vi "read_pbot_temperature.vi"(11 "Equip_Data":T1 {"h5File_refOut" format="%.0x"; "h5File_dsetOut" format="%.0x"}) -> (0 "error out":errorcluster, 3 "Temperature":dbl)   [LabVIEW 2015]
uses:
  controls/Equip_Data.ctl
  <vilib>/Utility/miscctls.llb/LV3DPointTypeDef.ctl
  controls/startScanData.ctl
  controls/scanInstrumentInfo.ctl
  <vilib>/addons/h5labview2/base/hid_t.ctl
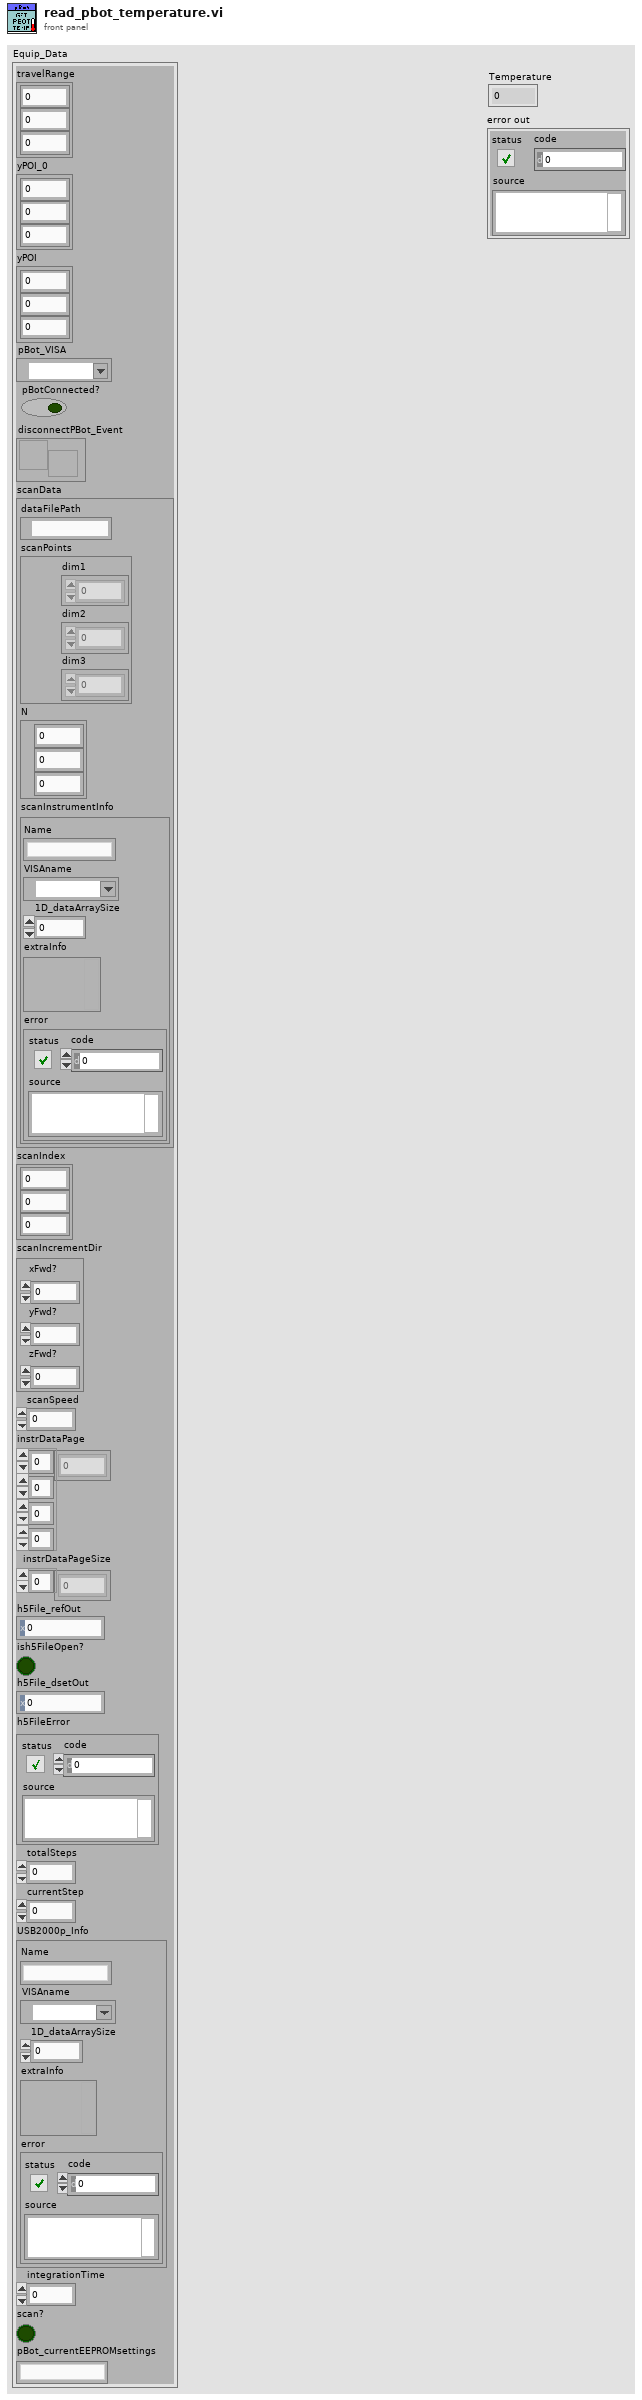
[diagram p1: front panel]
types:
  T1 = typedef "Equip_Data.ctl" = cluster{"travelRange":T2, "yPOI_0":T2, "yPOI":T2, "pBot_VISA":refnum<visa-resource-name>, "pBotConnected?":bool, "disconnectPBot_Event":refnum<user-event>, "scanData":T3, "scanIndex":cluster{"X":u16, "Y":u16, "Z":u16}, "scanIncrementDir":cluster{"xFwd?":i16, "yFwd?":i16, "zFwd?":i16}, "scanSpeed":u16, "instrDataPage":dbl[][][][], "instrDataPageSize":i32[], "h5File_refOut":T5, "ish5FileOpen?":bool, "h5File_dsetOut":T5, "h5FileError":errorcluster, "totalSteps":u32, "currentStep":u32, "USB2000p_Info":T4, "integrationTime":u32, "scan?":bool, "pBot_currentEEPROMsettings":string}
  T2 = typedef "LV3DPointTypeDef.ctl" = cluster{"X":sgl, "Y":sgl, "Z":sgl}
  T3 = typedef "startScanData.ctl" = cluster{"dataFilePath":path, "scanPoints":cluster{"dim1":sgl[], "dim2":sgl[], "dim3":sgl[]}, "N":cluster{"X":u16, "Y":u16, "Z":u16}, "scanInstrumentInfo":T4}
  T4 = typedef "scanInstrumentInfo.ctl" = cluster{"Name":string, "VISAname":refnum<visa-resource-name>, "1D_dataArraySize":u16, "extraInfo":variant, "error":errorcluster}
  T5 = typedef "hid_t.ctl" = i32
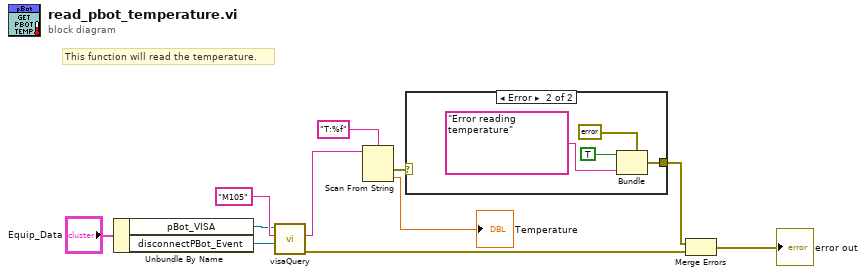
[diagram p0: block diagram]
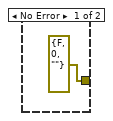
[diagram p2: hidden frame]
diagram:
  # "This function will read the temperature."
  n1 = Unbundle By Name("Equip_Data") -> ("pBot_VISA"=w1:refnum<visa-resource-name>, "disconnectPBot_Event"=w2:refnum<user-event>)
  n2 = call "visaQuery.vi"("disconnectPBot_Event"=w2, "stringToWrite"="M105" ("format string"), "VISA resource name"=w1) -> ("error Out"=w11:errorcluster, "String"=w8:string)  [unwired: 6 in, 1 out]
  n3 = Scan From String(format string="T:%f", input string=w8) -> (error out=w9:errorcluster, output 1=→"Temperature":dbl)  [unwired: 3 in, 2 out]
  n4 = case shown="Error" w9 {
    tunnel: [errorcluster {"status"=FALSE, "code"=0, "source"=""} ("error constant") w14] -> w10
    frame No Error {
    }
    frame Error {
      n5 = Bundle(cluster=errorcluster {"status"=TRUE, "code"=0, "source"=""} ("error constant"), "status"=TRUE, "source"="Error reading temperature" ("format string")) -> (w14:errorcluster)  [unwired: 1 in]
    }
  }
  n6 = Merge Errors(w10, w11) -> (→"error out":errorcluster)
